vi "Write States.vi"(8 "error in (no error)":errorcluster, 10 "States":T1, 11 "AttackerAimGoalTactic in":refnum<class "AttackerAimGoalTactic.lvclass">) -> (0 "error out":errorcluster, 3 "AttackerAimGoalTactic out":refnum<class "AttackerAimGoalTactic.lvclass">)   [LabVIEW 2018, in "AttackerAimGoalTactic.lvclass"]
uses:
  AttackerAimGoalTactic.lvclass
  States.ctl
  AttackerAimGoalTactic.lvclass/AttackerAimGoalTactic.ctl
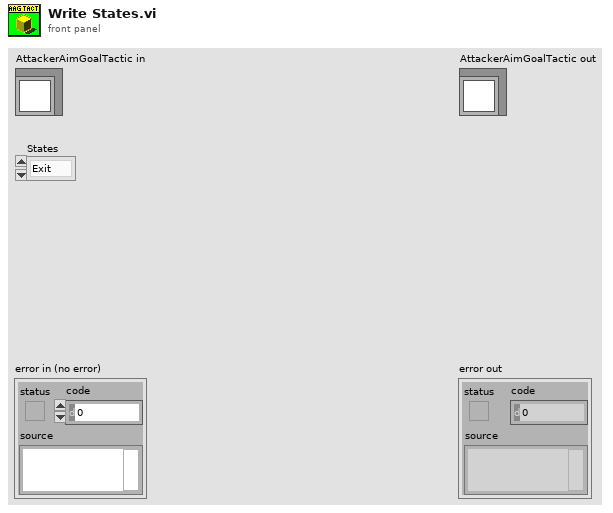
[diagram p1: front panel]
types:
  T1 = typedef "AttackerAimGoalTactic.lvclass/States.ctl" = enum16{"Exit", "AimGoal"}
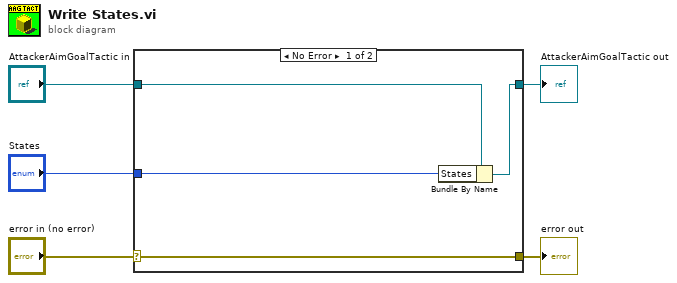
[diagram p0: block diagram]
diagram:
  n1 = case shown="No Error" "error in (no error)" {
    selector: "error in (no error)" -> [w9 w10]
    tunnel: [w9 w10] -> w4
    tunnel: [w7 w11] -> w2
    tunnel: "AttackerAimGoalTactic in" -> [w8 w11]
    tunnel: "States" -> [w6 _]
    frame No Error {
      n2 = Bundle By Name(cluster=w8, "States"=w6) -> (w7:refnum<class "AttackerAimGoalTactic.lvclass">)
    }
    frame Error {
    }
  }
  "error out" <- w4
  "AttackerAimGoalTactic out" <- w2
